vi "Basic Example.vi"() -> ()   [LabVIEW 2013, in "Progress Bar.lvlib"]
uses:
  <vilib>/NI/Progress Bar/Progress Bar.lvlib
  <vilib>/NI/Progress Bar/Controls/Update Bar Actions.ctl
  <vilib>/NI/Progress Bar/Controls/Progress Bar Properties.ctl
panel:
  out "exists?":bool
  out "error out":errorcluster
  # "A progress bar appears as a separate window. \nExample returns errors generated by the progress bar API., even though\nany progress bar errors should be ignored in the final application."
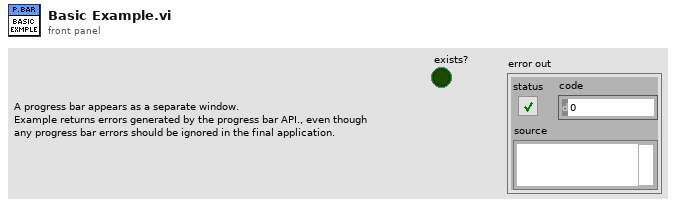
[diagram p1: front panel]
types:
  T1 = typedef "Progress Bar.lvlib/Progress Bar Properties.ctl" = cluster{"Background Color":u32, "Installer Title":string, "Title Color":u32, "Action Text":string, "Text Color":u32, "Slider Value":u8, "Bar Color":u32, "Timeout":i32}
  T2 = typedef "Progress Bar.lvlib/Update Bar Actions.ctl" = enum16{"Add To Existing", "Set to Value"}
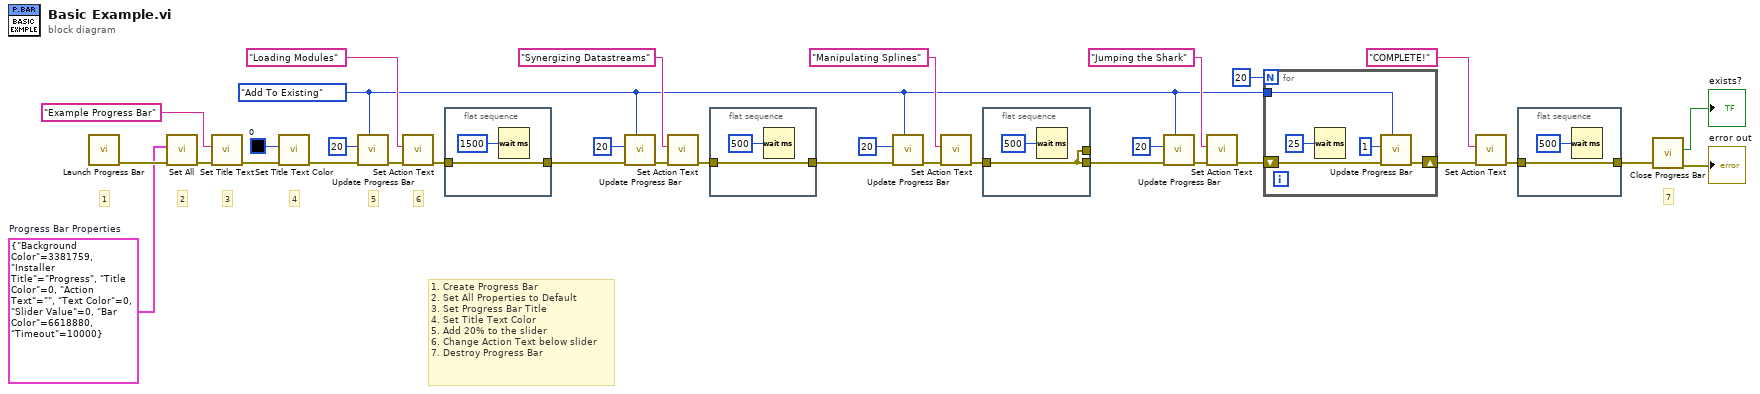
[diagram p0: block diagram]
diagram:
  w6 = T1 {"Background Color"=3381759, "Installer Title"="Progress", "Title Color"=0, "Action Text"="", "Text Color"=0, "Slider Value"=0, "Bar Color"=6618880, "Timeout"=10000}  # Progress Bar Properties
  w5 = Update_Bar_Actions."Add To Existing" ("Action")
  # "7"
  # "6"
  # "5"
  # "4"
  # "3"
  # "2"
  # "1"
  # "1. Create Progress Bar\n2. Set All Properties to Default\n3. Set Progress Bar Title\n4. Set Title Text Color\n5. Add 20% to the slider\n6. Change Action Text below slider\n7. Destroy Progress Bar"
  n1 = call <vilib>:"Launch Progress Bar.vi"() -> ("error out"=w7:errorcluster)  [unwired: 10 in, 1 out]
  n2 = call <vilib>:"Set All.vi"("error in (no error)"=w7, "Progress Bar Properties (Default)"=w6) -> ("error out"=w30:errorcluster)  [unwired: 9 in]
  n3 = call <vilib>:"Set Title Text.vi"("error in (no error)"=w30, "Installer Title"="Example Progress Bar") -> ("error out"=w33:errorcluster)  [unwired: 9 in]
  n4 = call <vilib>:"Set Title Text Color.vi"("error in (no error)"=w33, "Color Box"=u32 0) -> ("error out"=w29:errorcluster)  [unwired: 9 in]
  n5 = call <vilib>:"Update Progress Bar.vi"("Action"=w5, "error in (no error)"=w29, "Value"=u8 20) -> ("error out"=w28:errorcluster)  [unwired: 8 in]
  n6 = call <vilib>:"Set Action Text.vi"("error in (no error)"=w28, "Action Text"="Loading Modules") -> ("error out"=w27:errorcluster)  [unwired: 9 in]
  n7 = flat-sequence {
    tunnel: w27 -> [w35]
    tunnel: [w35] -> w14
    frame #0 {
      n8 = Wait (ms)(milliseconds to wait=u32 1500) -> ()  [unwired: 1 out]
    }
  }
  n9 = call <vilib>:"Update Progress Bar.vi"("Action"=w5, "error in (no error)"=w14, "Value"=u8 20) -> ("error out"=w24:errorcluster)  [unwired: 8 in]
  n10 = call <vilib>:"Set Action Text.vi"("error in (no error)"=w24, "Action Text"="Synergizing Datastreams") -> ("error out"=w23:errorcluster)  [unwired: 9 in]
  n11 = flat-sequence {
    tunnel: w23 -> [w37]
    tunnel: [w37] -> w13
    frame #0 {
      n12 = Wait (ms)(milliseconds to wait=u32 500) -> ()  [unwired: 1 out]
    }
  }
  n13 = call <vilib>:"Update Progress Bar.vi"("Action"=w5, "error in (no error)"=w13, "Value"=u8 20) -> ("error out"=w20:errorcluster)  [unwired: 8 in]
  n14 = call <vilib>:"Set Action Text.vi"("error in (no error)"=w20, "Action Text"="Manipulating Splines") -> ("error out"=w19:errorcluster)  [unwired: 9 in]
  n15 = flat-sequence {
    tunnel: w19 -> [w39]
    tunnel: [w39] -> _
    tunnel: [w39] -> w12
    frame #0 {
      n16 = Wait (ms)(milliseconds to wait=u32 500) -> ()  [unwired: 1 out]
    }
  }
  n17 = call <vilib>:"Update Progress Bar.vi"("Action"=w5, "error in (no error)"=w12, "Value"=u8 20) -> ("error out"=w16:errorcluster)  [unwired: 8 in]
  n18 = call <vilib>:"Set Action Text.vi"("error in (no error)"=w16, "Action Text"="Jumping the Shark") -> ("error out"=w3:errorcluster)  [unwired: 9 in]
  n19 = for {
    N: 20 ("Value") -> [_]
    tunnel: w5 -> [w42]
    shift-right: [w45] -> w11
    shift-left: w3 -> [w44]
    n20 = Wait (ms)(milliseconds to wait=u32 25) -> ()  [unwired: 1 out]
    n21 = call <vilib>:"Update Progress Bar.vi"("Action"=w42, "error in (no error)"=w44, "Value"=u8 1) -> ("error out"=w45:errorcluster)  [unwired: 8 in]
  }
  n22 = call <vilib>:"Set Action Text.vi"("error in (no error)"=w11, "Action Text"="COMPLETE!") -> ("error out"=w10:errorcluster)  [unwired: 9 in]
  n23 = flat-sequence {
    tunnel: w10 -> [w46]
    tunnel: [w46] -> w8
    frame #0 {
      n24 = Wait (ms)(milliseconds to wait=u32 500) -> ()  [unwired: 1 out]
    }
  }
  n25 = call <vilib>:"Close Progress Bar.vi"("error in (no error)"=w8) -> ("error out"=→"error out":errorcluster, "exists?"=→"exists?":bool)  [unwired: 9 in]
